vi "MyrioProject.vi"() -> ()   [LabVIEW 2018]
doc: "The myRIO Project template acquires acceleration data from the onboard accelerometer and displays the changes of acceleration values in a waveform chart."
uses:
  <vilib>/Platform/TimedLoop/XDataNode/timing_clust.ctl
  <vilib>/Platform/TimedLoop/XDataNode/nitl_modes.ctl
  <vilib>/Platform/TimedLoop/XDataNode/wakeup.ctl
  <vilib>/myRIO/Common/Instrument Driver Framework/myRIO v1.0/Encoder/typedefs/Encoder Signal Mode.ctl
  <vilib>/Analysis/Matrix/Datatypes/RealMatrix.ctl
  <vilib>/myRIO/Instrument Drivers/Onboard IO/PWM/typedefs/PWM Reference.ctl
  <vilib>/myRIO/Common/Instrument Driver Framework/Utilities/typedefs/myRIO Generic Hardware Reference.ctl
  <vilib>/myRIO/Common/Instrument Driver Framework/Utilities/typedefs/Hardware Version Enum.ctl
  <vilib>/myRIO/Common/Instrument Driver Framework/Utilities/typedefs/myRIO v1.0 Reference.ctl
  <vilib>/myRIO/Common/Instrument Driver Framework/Utilities/typedefs/Generic FPGA Reference.ctl
  <vilib>/myRIO/Common/Instrument Driver Framework/myRIO v1.0/PWM/typedefs/PWM Channels Enum.ctl
  <vilib>/myRIO/Instrument Drivers/Onboard IO/PWM/typedefs/PWM Configuration.ctl
  <vilib>/userdefined/High Color/nirio_resource_hc.ctl
  <vilib>/myRIO/Common/Instrument Driver Framework/myRIO v1.0/Encoder/typedefs/Encoder Configuration v1.0.ctl
  <vilib>/myRIO/Instrument Drivers/Onboard IO/Encoder/typedefs/Encoder Reference.ctl
  <vilib>/myRIO/Common/Instrument Driver Framework/myRIO v1.0/Encoder/typedefs/Encoder Channels Enum.ctl
  <vilib>/myRIO/Instrument Drivers/Onboard IO/DIO/typedefs/DIO Reference.ctl
  <vilib>/myRIO/Common/Instrument Driver Framework/myRIO v1.0/DIO/typedefs/DIO Channels List.ctl
  <vilib>/myRIO/Common/Instrument Driver Framework/myRIO v1.0/DIO/typedefs/DIO Channels Enum.ctl
  <vilib>/myRIO/Instrument Drivers/Onboard IO/AI/typedefs/AI Reference.ctl
  <vilib>/myRIO/Common/Instrument Driver Framework/myRIO v1.0/AI/typedefs/AI Channels List.ctl
  <vilib>/myRIO/Common/Instrument Driver Framework/myRIO v1.0/AI/typedefs/AI Channels Enum.ctl
  <vilib>/myRIO/Common/Instrument Driver Framework/Utilities/typedefs/Analog Scaling Constants List.ctl
  <vilib>/myRIO/Common/Instrument Driver Framework/Utilities/typedefs/Analog Scaling Constants.ctl
  <vilib>/myRIO/Common/Instrument Driver Framework/myRIO v1.0/PWM/vis/myRIO v1.1 Open PWM.vi
  <vilib>/myRIO/Common/Instrument Driver Framework/myRIO v1.0/Encoder/vis/myRIO v1.1 Open Encoder.vi
  <vilib>/myRIO/Common/Instrument Driver Framework/Utilities/vis/Is FPGA Ref Available.vi
  <vilib>/myRIO/Common/Instrument Driver Framework/myRIO v1.0/AI/vis/myRIO v1.1 Open AI.vi
  <vilib>/myRIO/Common/Instrument Driver Framework/myRIO v1.0/DIO/vis/myRIO v1.1 Open DIO.vi
  <vilib>/myRIO/Instrument Drivers/Onboard IO/PWM/vis/Set Duty Cycle and Frequency.vi
  <vilib>/myRIO/Instrument Drivers/Onboard IO/DIO/vis/Write.vi
  <vilib>/myRIO/Common/Instrument Driver Framework/Utilities/vis/Validate Channels.vi
  <vilib>/myRIO/Common/Instrument Driver Framework/myRIO v1.0/PWM/vis/myRIO v1.0 Reserve PWM.vi
  <vilib>/myRIO/Common/Instrument Driver Framework/myRIO v1.0/Encoder/vis/myRIO v1.0 Reserve Encoder.vi
  <vilib>/myRIO/Common/Instrument Driver Framework/myRIO v1.0/AI/vis/myRIO v1.0 Reserve AI.vi
  <vilib>/myRIO/Common/Instrument Driver Framework/myRIO v1.0/DIO/vis/myRIO v1.0 Reserve DIO.vi
  <vilib>/myRIO/Common/Instrument Driver Framework/myRIO v1.0/Encoder/vis/myRIO v1.0 Close Encoder.vi
  <vilib>/myRIO/Common/Instrument Driver Framework/myRIO v1.0/PWM/vis/myRIO v1.0 Close PWM.vi
  <vilib>/myRIO/Common/Instrument Driver Framework/myRIO v1.0/PWM/vis/myRIO v1.0 Build MUX Configuration PWM.vi
  <vilib>/myRIO/Common/Instrument Driver Framework/myRIO v1.0/Resource Manager/vis/myRIO v1.0 Reserve Channel List.vi
  <vilib>/myRIO/Common/Instrument Driver Framework/myRIO v1.0/Encoder/vis/myRIO v1.0 Build MUX Configuration Encoder.vi
  <vilib>/myRIO/Common/Instrument Driver Framework/myRIO v1.0/AI/vis/myRIO v1.0 Build MUX Configuration AI.vi
  <vilib>/myRIO/Common/Instrument Driver Framework/myRIO v1.0/DIO/vis/myRIO v1.0 Build MUX Configuration DIO.vi
  <vilib>/myRIO/Common/Instrument Driver Framework/myRIO v1.0/Encoder/vis/myRIO v1.0 Unreserve Encoder.vi
  <vilib>/myRIO/Common/Instrument Driver Framework/myRIO v1.0/PWM/vis/myRIO v1.0 Unreserve PWM.vi
  <vilib>/myRIO/Common/Instrument Driver Framework/myRIO v1.0/Resource Manager/vis/myRIO v1.0 Create Configuration List.vi
  <vilib>/myRIO/Common/Instrument Driver Framework/myRIO v1.0/Resource Manager/vis/myRIO v1.0 Reserve Channel.vi
  <vilib>/myRIO/Common/Instrument Driver Framework/myRIO v1.0/Resource Manager/vis/myRIO v1.0 Unreserve Channel.vi
  <vilib>/myRIO/Common/Instrument Driver Framework/myRIO v1.0/Resource Manager/vis/myRIO v1.0 Unreserve Channel List.vi
  <vilib>/myRIO/Common/Instrument Driver Framework/myRIO v1.0/Resource Manager/vis/myRIO v1.0 Build Mutex Name.vi
  <vilib>/Utility/VariantDataType/GetNumericInfo.vi
  <vilib>/Utility/error.llb/Error Cluster From Error Code.vi
  <vilib>/myRIO/Common/Instrument Driver Framework/myRIO v1.0/myRIO v1.1 Open.vi
  <vilib>/myRIO/Common/Instrument Driver Framework/Utilities/vis/IO Manager.vi
  <vilib>/myRIO/Common/Instrument Driver Framework/Utilities/vis/Configuration Manager.vi
  <vilib>/myRIO/Common/Instrument Driver Framework/myRIO v1.0/Resource Manager/vis/myRIO v1.0 Configure IO.vi
  <vilib>/myRIO/Common/Instrument Driver Framework/myRIO v1.0/myRIO v1.0 Close.vi
  <vilib>/myRIO/Common/Instrument Driver Framework/myRIO v1.0/PWM/vis/myRIO v1.0 Write PWM.vi
  <vilib>/myRIO/Common/Instrument Driver Framework/myRIO v1.0/Encoder/vis/myRIO v1.0 Configure Encoder.vi
  <vilib>/myRIO/Common/Instrument Driver Framework/myRIO v1.0/Encoder/vis/myRIO v1.0 Enable Encoder.vi
  <vilib>/myRIO/Common/Instrument Driver Framework/myRIO v1.0/DIO/vis/myRIO v1.0 Read DIO.vi
  <vilib>/myRIO/Common/Instrument Driver Framework/myRIO v1.0/AI/vis/myRIO v1.0 Get Scaling Constants AI.vi
  <vilib>/myRIO/Common/Instrument Driver Framework/myRIO v1.0/AI/vis/myRIO v1.0 Read AI.vi
  <vilib>/myRIO/Common/Instrument Driver Framework/myRIO v1.0/Encoder/vis/myRIO v1.0 Read Encoder.vi
  <vilib>/myRIO/Common/Instrument Driver Framework/myRIO v1.0/DIO/vis/myRIO v1.0 Write DIO.vi
  <vilib>/myRIO/Common/Instrument Driver Framework/myRIO v1.0/Encoder/vis/myRIO v1.0 Shutdown Encoder.vi
  <vilib>/myRIO/Common/Instrument Driver Framework/myRIO v1.0/PWM/vis/myRIO v1.0 Shutdown PWM.vi
  <vilib>/platform/TimedLoop/XDataNode/XDataNode.xnode
  <vilib>/myRIO/Instrument Drivers/Onboard IO/PWM/vis/myRIO PWM Open.xnode
  <vilib>/myRIO/Instrument Drivers/Onboard IO/Encoder/vis/myRIO Encoder Open.xnode
  <vilib>/myRIO/Express VI/Onboard IO/PWM/PWM Express VI.xnode
  <vilib>/myRIO/Express VI/Onboard Devices/Button/Button Express VI.xnode
  <vilib>/myRIO/Instrument Drivers/Onboard IO/DIO/vis/myRIO DIO Open.xnode
  <vilib>/myRIO/Express VI/Onboard IO/AI/AI Express VI.xnode
  <vilib>/myRIO/Instrument Drivers/Onboard IO/AI/vis/myRIO AI Open.xnode
  <vilib>/myRIO/Express VI/Onboard IO/DO/DO Express VI.xnode
  <vilib>/Platform/TimedLoop/XDataNode/XDNodeRunTimeDep.lvlib
  <vilib>/myRIO/Instrument Drivers/Onboard IO/Encoder/Encoder.lvlib
  <vilib>/myRIO/Instrument Drivers/Onboard IO/PWM/PWM.lvlib
  <vilib>/myRIO/Instrument Drivers/Onboard IO/DIO/DIO.lvlib
  <vilib>/myRIO/Instrument Drivers/Onboard IO/AI/AI.lvlib
  <vilib>/Analysis/Matrix/NI_Matrix.lvlib
panel:
  out "data":dbl
  out "Double 2":dbl
  out "Double":dbl
  out "sensor2 (A/AI2 (Pin 7))":dbl
  out "sensor1":dbl
  out "stallRojo (A/AI0 (Pin 3))":dbl
  out "stallBlanco (A/AI1 (Pin 5))":dbl
  in  "MANUAL 2":bool
  in  "Stop Button":bool
  in  "Start":bool
  out "element":dbl
  out "element 2":dbl
  out "subarray 2":dbl[][](array[numeric])
  out "subarray":dbl[][](array[numeric])
  out "vectores":dbl[][][](array[numeric])
  in  "saturacion":dbl=0.3
  in  "Duty Cycle 2":dbl(slide)=0.5 scale=0.05..0.1
  in  "Duty Cycle":dbl(slide)=0.5 scale=0.05..0.1
  in  "Reset Counter 2":bool
  in  "Reset Counter":bool
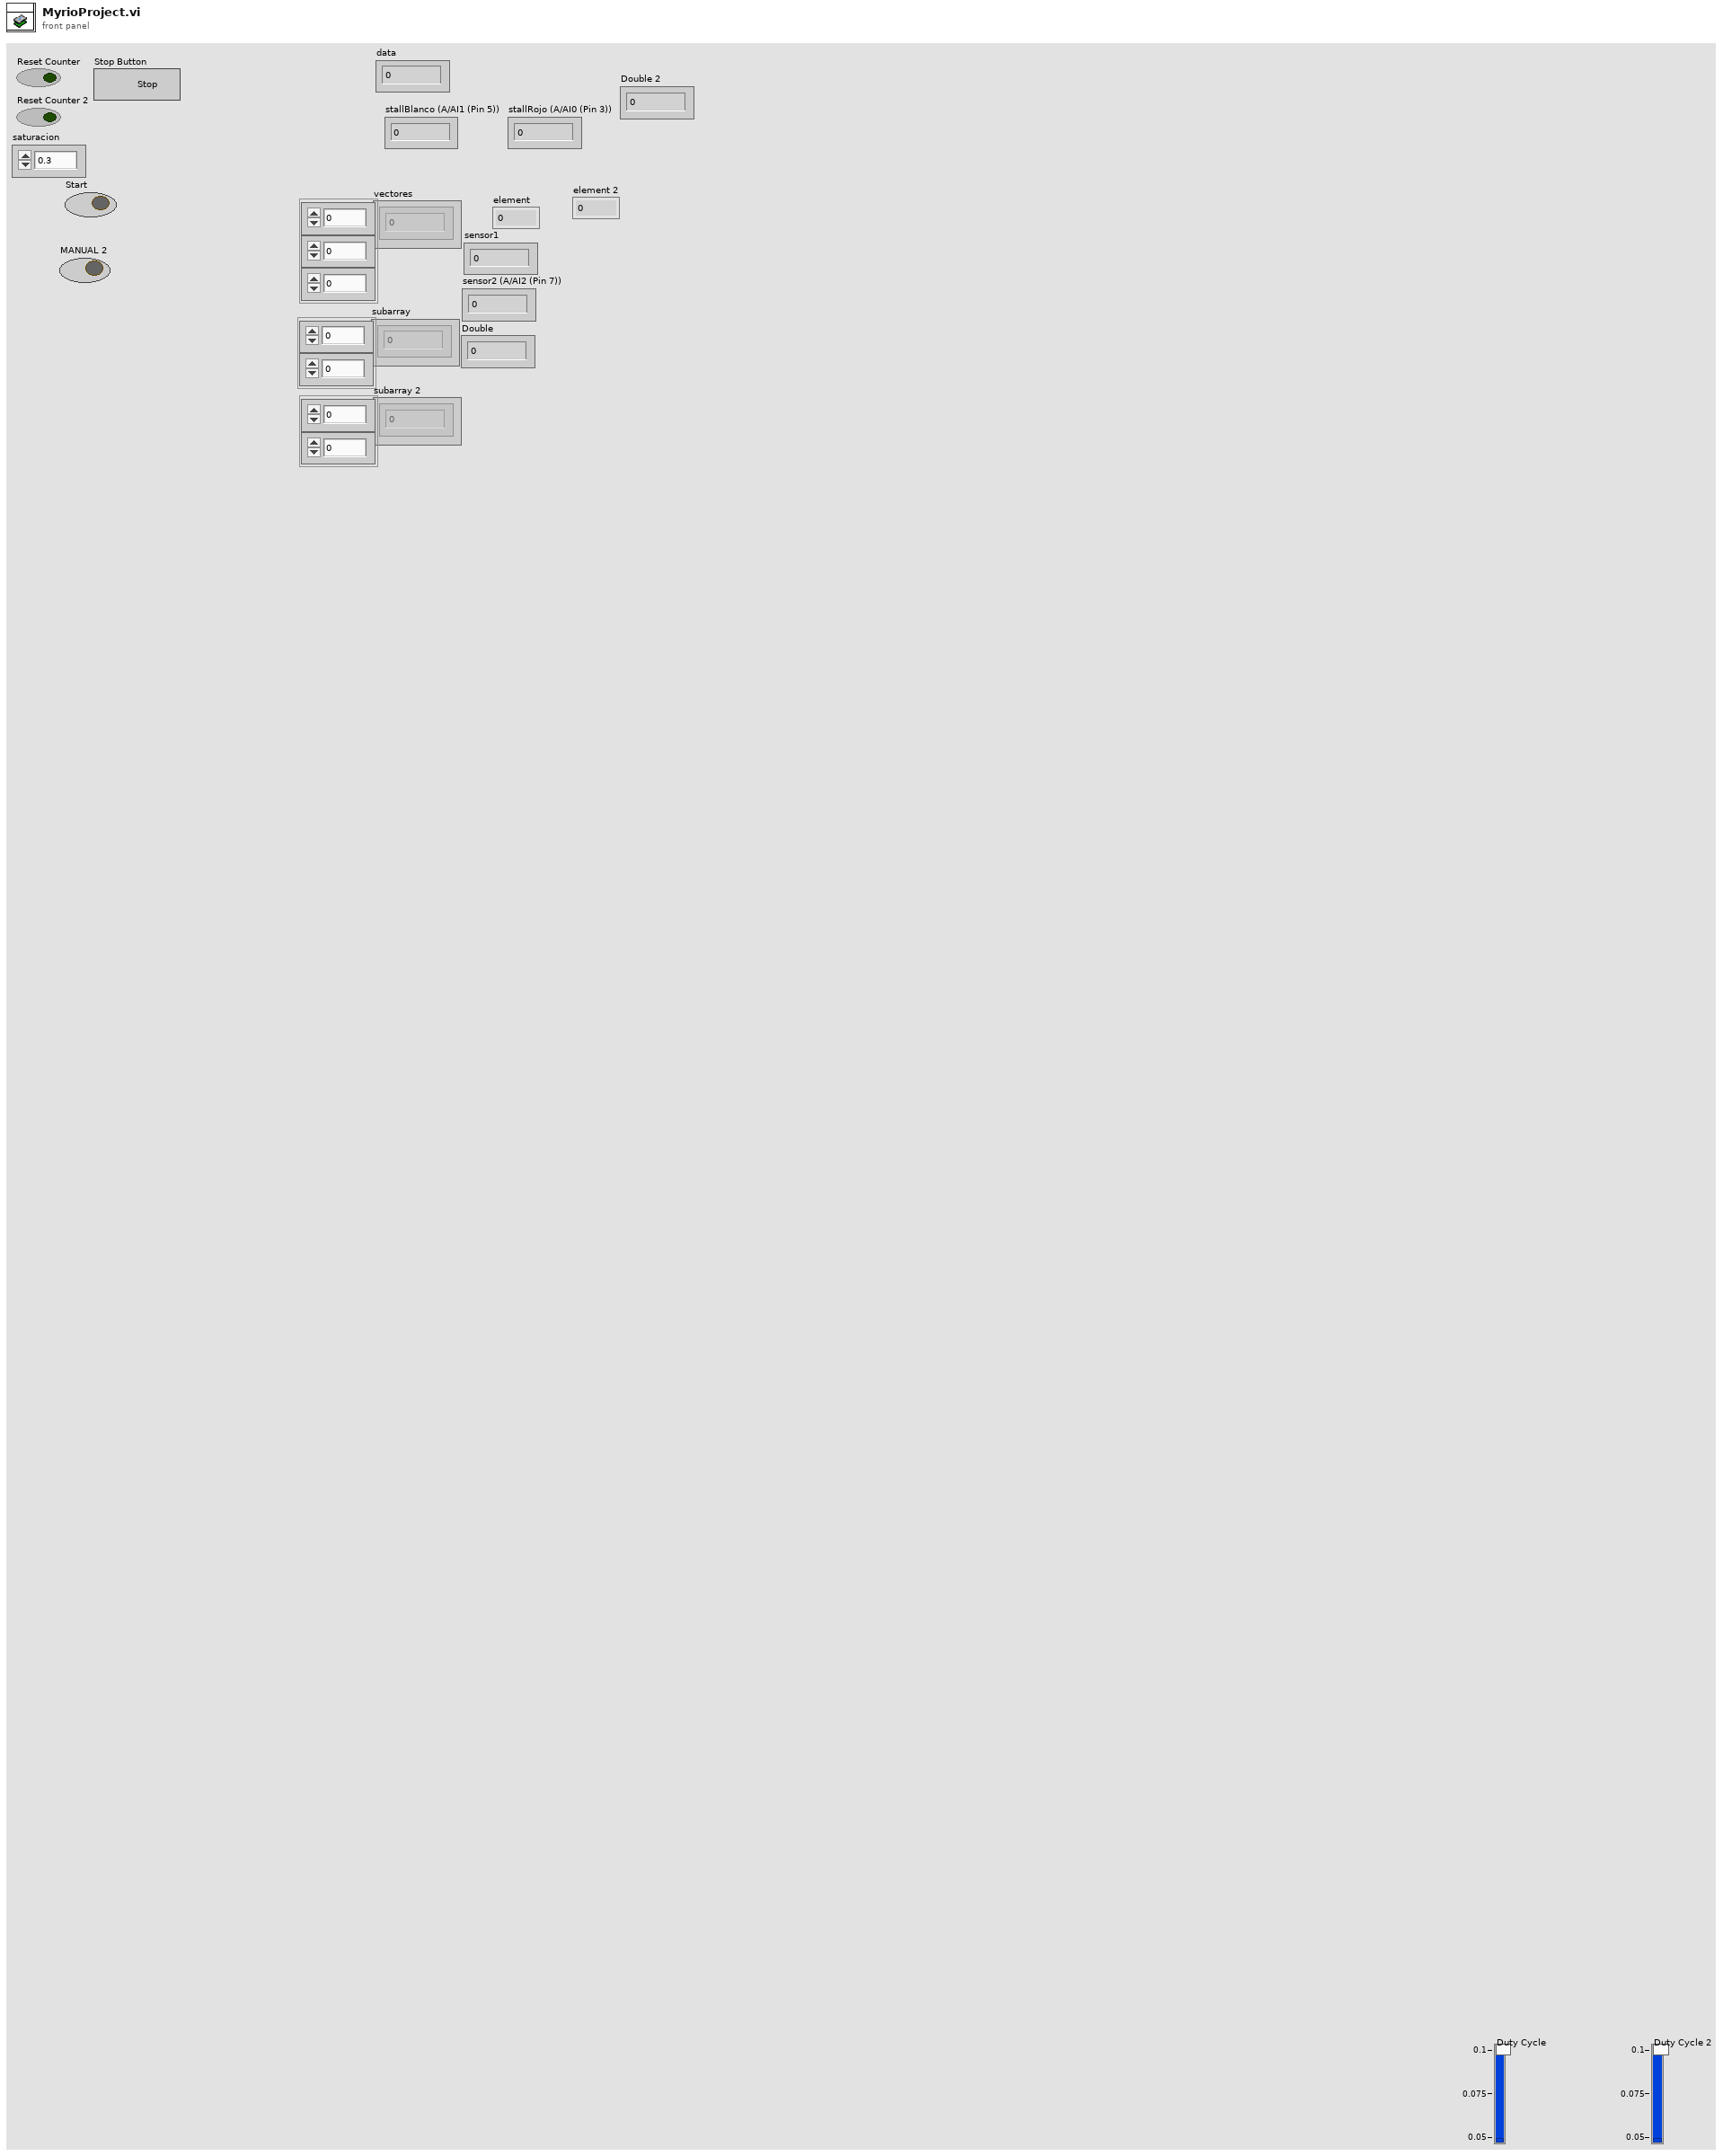
[diagram p1: front panel]
types:
  T1 = typedef "NI_Matrix.lvlib/RealMatrix.ctl" = dbl[][]
  T2 = typedef "Encoder Signal Mode.ctl" = enum16{"Quadrature phase signal", "Step and direction signal"}
  T3 = typedef "PWM.lvlib/PWM Reference.ctl" = cluster{"myRIO Reference":T4, "PWM Channels Enum":T8, "PWM Configuration":T9}
  T4 = typedef "myRIO Generic Hardware Reference.ctl" = cluster{"myRIO Model":T5, "myRIO Hardware Reference":T6}
  T5 = typedef "Hardware Version Enum.ctl" = enum16{"Unknown", "myRIO-1900", "myRIO-1950", "roboRIO", "NI ELVIS RIO CM", "ELVIS III"}
  T6 = typedef "myRIO v1.0 Reference.ctl" = cluster{"Generic FPGA Reference":T7, "Allow multiple opens":bool}
  T7 = typedef "Generic FPGA Reference.ctl" = refnum<k20>
  T8 = typedef "PWM Channels Enum.ctl" = enum16{"Not Connected", "C/PWM0", "C/PWM1", "A/PWM0", "A/PWM1", "A/PWM2", "A/PWM3", "A/PWM4", "A/PWM5", "A/PWM6", "A/PWM7", "A/PWM8", "A/PWM9", "A/PWM10", "A/PWM11", "A/PWM12", "A/PWM13", "A/PWM14", "A/PWM15", "A/PWM16", "A/PWM17", "A/PWM18", "A/PWM19", "B/PWM0", "B/PWM1", "B/PWM2", "B/PWM3", "B/PWM4", "B/PWM5", "B/PWM6", "B/PWM7", "B/PWM8", "B/PWM9", "B/PWM10", "B/PWM11", "B/PWM12", "B/PWM13", "B/PWM14", "B/PWM15", "B/PWM16", "B/PWM17", "B/PWM18", "B/PWM19", "PWM/PWM0", "PWM/PWM1", "PWM/PWM2", "PWM/PWM3", "PWM/PWM4", "PWM/PWM5", "PWM/PWM6", "PWM/PWM7", "PWM/PWM8", "PWM/PWM9"}
  T9 = typedef "PWM.lvlib/PWM Configuration.ctl" = cluster{"Frequency":dbl, "Duty Cycle":dbl}
  T10 = typedef "Encoder.lvlib/Encoder Reference.ctl" = cluster{"myRIO Reference":T4, "Encoder Channels Enum":T11}
  T11 = typedef "Encoder Channels Enum.ctl" = enum16{"Not Connected", "C/ENC0", "C/ENC1", "A/ENC", "A/ENC0", "A/ENC1", "A/ENC2", "A/ENC3", "A/ENC4", "A/ENC5", "A/ENC6", "A/ENC7", "A/ENC8", "A/ENC9", "B/ENC", "B/ENC0", "B/ENC1", "B/ENC2", "B/ENC3", "B/ENC4", "B/ENC5", "B/ENC6", "B/ENC7", "B/ENC8", "B/ENC9", "DIO/ENC0", "DIO/ENC1", "DIO/ENC2", "DIO/ENC3", "DIO/ENC4"}
  T12 = typedef "XDNodeRunTimeDep.lvlib/timing_clust.ctl" = cluster{"Expected End [f-1]":u64, "Actual End [f-1]":u64, "Finished Late? [f-1]":bool, "Expected End [i-1]":u64, "Actual End [i-1]":u64, "Finished Late? [i-1]":bool, "Expected Start [i]":u64, "Actual Start [i]":u64, "Expected Start [f]":u64, "Actual Start [f]":u64, "Source Name":string, "Structure Name":string, "Period":i64, "Deadline":i64, "Offset":i64, "Start":i64, "Priority":i32, "Timeout":i32, "Mode":T13, "Wakeup Reason":T14, "Error":errorcluster, "Source Type":string, "Secondary Source Type":string, "Global End Time":u64, "Global Start Time":u64, "Frame Duration":u64, "Iteration Duration":u64, "Assigned CPU":i32, "I/O Scan Engine Mode":u32}
  T13 = typedef "XDNodeRunTimeDep.lvlib/nitl_modes.ctl" = enum32{"No Change", "Process missed periods, maintain original phase", "Discard missed periods, maintain original phase", "Process missed periods, ignore original phase", "Discard missed periods, ignore original phase"}
  T14 = typedef "XDNodeRunTimeDep.lvlib/wakeup.ctl" = enum32{"Normal", "Aborted", "Asynchronous wakeup", "Timing source error", "Timed loop error", "Timeout"}
  T15 = enum16{"normal", "grande-Sensor", "grande home", "peque-sensor", "peque- home", "peque-reset"}
  T16 = typedef "nirio_resource_hc.ctl" = tag
  T17 = typedef "AI.lvlib/AI Reference.ctl" = cluster{"myRIO Reference":T4, "AI Channels List":T18, "AI Scaling Constants List":T20}
  T18 = typedef "AI Channels List.ctl" = T19[]
  T19 = typedef "AI Channels Enum.ctl" = enum16{"Not Connected", "AudioIn/Left", "AudioIn/Right", "C/AI0", "C/AI1", "A/AI0", "A/AI1", "A/AI2", "A/AI3", "A/AI4", "A/AI5", "A/AI6", "A/AI7", "B/AI0", "B/AI1", "B/AI2", "B/AI3", "B/AI4", "B/AI5", "B/AI6", "B/AI7", "AI/AI0", "AI/AI1", "AI/AI2", "AI/AI3", "A/AI0 (DIFF)", "A/AI1 (DIFF)", "A/AI2 (DIFF)", "A/AI3 (DIFF)", "B/AI0 (DIFF)", "B/AI1 (DIFF)", "B/AI2 (DIFF)", "B/AI3 (DIFF)"}
  T20 = typedef "Analog Scaling Constants List.ctl" = T21[]
  T21 = typedef "Analog Scaling Constants.ctl" = cluster{"LSB Weight (Volts)":dbl, "Offset (Volts)":dbl, "Signed?":bool}
  T22 = typedef "DIO.lvlib/DIO Reference.ctl" = cluster{"myRIO Reference":T4, "DIO Channels List":T23}
  T23 = typedef "DIO Channels List.ctl" = T24[]
  T24 = typedef "DIO Channels Enum.ctl" = enum16{"Not Connected", "C/DIO0", "C/DIO1", "C/DIO2", "C/DIO3", "C/DIO4", "C/DIO5", "C/DIO6", "C/DIO7", "A/DIO0", "A/DIO1", "A/DIO2", "A/DIO3", "A/DIO4", "A/DIO5", "A/DIO6", "A/DIO7", "A/DIO8", "A/DIO9", "A/DIO10", "A/DIO11", "A/DIO12", "A/DIO13", "A/DIO14", "A/DIO15", "A/DIO16", "A/DIO17", "A/DIO18", "A/DIO19", "B/DIO0", "B/DIO1", "B/DIO2", "B/DIO3", "B/DIO4", "B/DIO5", "B/DIO6", "B/DIO7", "B/DIO8", "B/DIO9", "B/DIO10", "B/DIO11", "B/DIO12", "B/DIO13", "B/DIO14", "B/DIO15", "B/DIO16", "B/DIO17", "B/DIO18", "B/DIO19", "LED0", "LED1", "LED2", "LED3", "Button0", "DIO/DIO0", "DIO/DIO1", "DIO/DIO2", "DIO/DIO3", "DIO/DIO4", "DIO/DIO5", "DIO/DIO6", "DIO/DIO7", "DIO/DIO8", "DIO/DIO9", "SPI/CS0", "SPI/CS1", "SPI/CS2", "SPI/CS3", "LED RADIO (Green)", "LED RADIO (Red)", "LED COMM (Green)", "LED COMM (Red)", "LED MODE (Green)", "LED MODE (Red)"}
  T25 = cluster{dbl, "saturacion":dbl, "Counter Value":i32, "seconds since 1Jan1904":timestamp, dbl, dbl, dbl}
  T26 = cluster{"Double":dbl, "dbl Scaled Value":dbl, "Output":dbl, "seconds since 1Jan1904":timestamp, dbl, dbl, dbl}
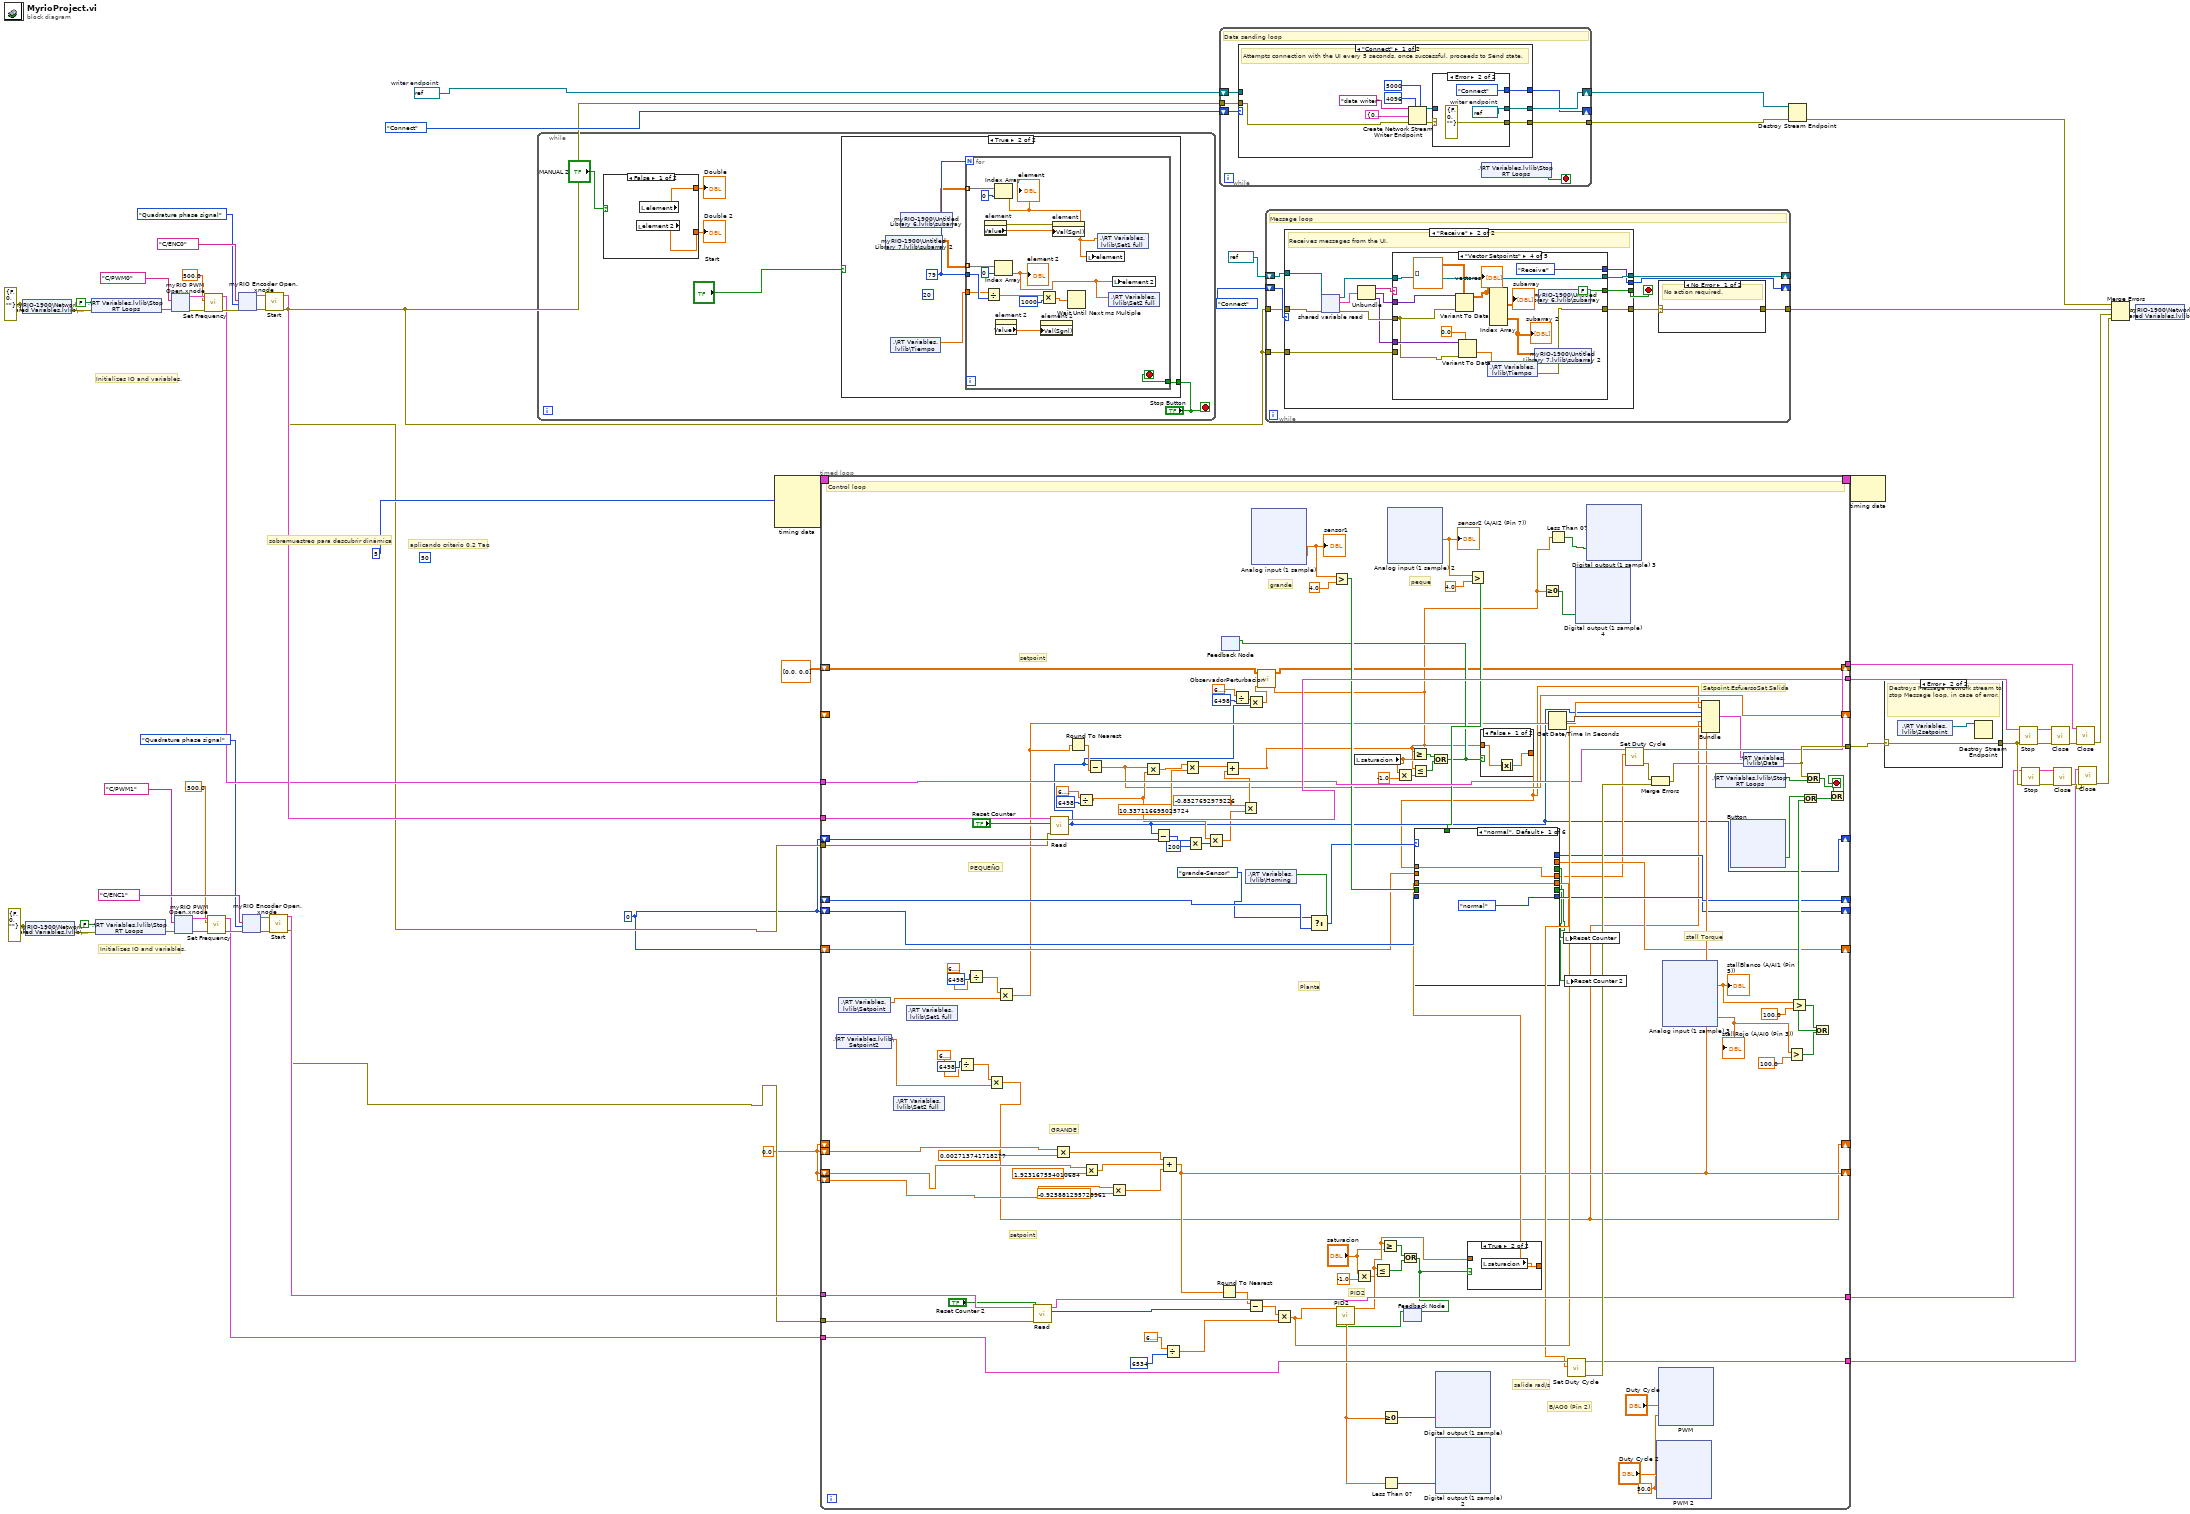
[diagram p0: block diagram]
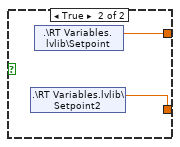
[diagram p2: hidden frame]
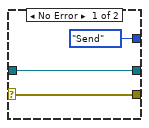
[diagram p5: hidden frame]
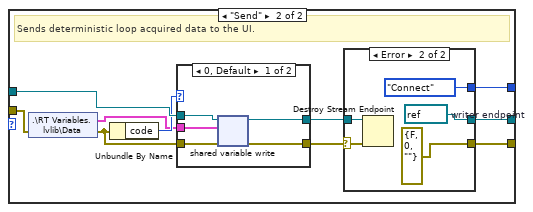
[diagram p6: hidden frame]
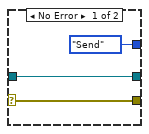
[diagram p7: hidden frame]
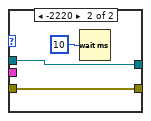
[diagram p8: hidden frame]
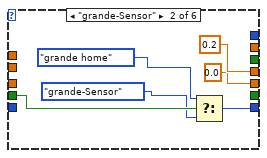
[diagram p9: hidden frame]
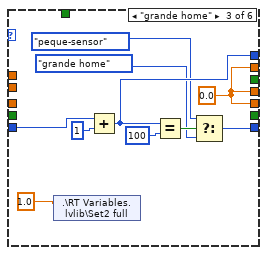
[diagram p10: hidden frame]
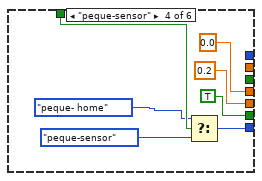
[diagram p11: hidden frame]
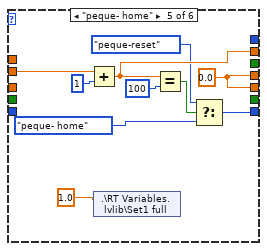
[diagram p12: hidden frame]
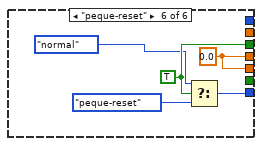
[diagram p13: hidden frame]
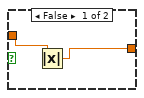
[diagram p14: hidden frame]
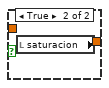
[diagram p15: hidden frame]
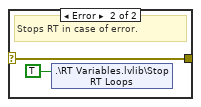
[diagram p16: hidden frame]
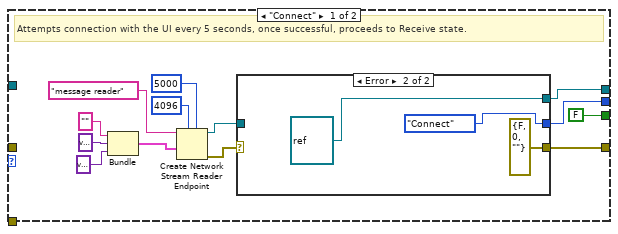
[diagram p17: hidden frame]
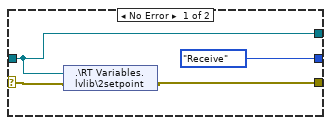
[diagram p18: hidden frame]
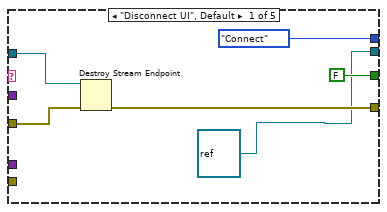
[diagram p19: hidden frame]
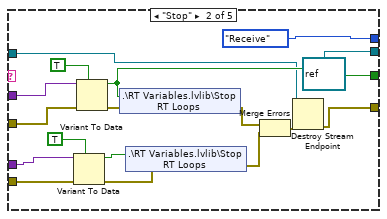
[diagram p20: hidden frame]
diagram:
  w2 = 0.0
  w3 = 0
  (unwired) 50
  w15 = refnum<k21> refnum  # writer endpoint
  w28 = errorcluster {"status"=FALSE, "code"=0, "source"=""} ("error IO")
  w50 = errorcluster {"status"=FALSE, "code"=0, "source"=""} ("error IO")
  # "aplicando criterio 0.2 Tao"
  # "sobremuestreo para descubrir dinámica"
  # "Initializes IO and variables."
  # "Initializes IO and variables."
  n1 = shared-variable "myRIO-1900\\Network Shared Variables.lvlib\\error IO"(w50, error in=w50) -> (error out=w51:errorcluster)
  n2 = shared-variable "myRIO-1900\\Network Shared Variables.lvlib\\error IO"(w28, error in=w28) -> (error out=w29:errorcluster)
  n3 = shared-variable ".\\RT Variables.lvlib\\Stop RT Loops"(FALSE ("Stop RT Loops"), error in=w51) -> (error out=w38:errorcluster)
  n4 = shared-variable ".\\RT Variables.lvlib\\Stop RT Loops"(FALSE ("Stop RT Loops"), error in=w29) -> (error out=w21:errorcluster)
  n5 = xnode "myRIO PWM Open.xnode"("error in (no error)"=w38, "Channel Name"=tag "C/PWM0") -> ("error out"=w40:errorcluster, "PWM Ref Out"=w39:T3)  [unwired: 1 in]
  n6 = xnode "myRIO PWM Open.xnode"("error in (no error)"=w21, "Channel Name"=tag "C/PWM1") -> ("error out"=w23:errorcluster, "PWM Ref Out"=w22:T3)  [unwired: 1 in]
  n7 = call <vilib>:"Set Frequency.vi"("error in (no error)"=w40, "Frequency [Hz]"=500.0, "PWM Ref In"=w39) -> ("error out"=w37:errorcluster, "PWM Ref Out"=w34:T3)  [unwired: 6 in]
  n8 = call <vilib>:"Set Frequency.vi"("error in (no error)"=w23, "Frequency [Hz]"=500.0, "PWM Ref In"=w22) -> ("error out"=w20:errorcluster, "PWM Ref Out"=w16:T3)  [unwired: 6 in]
  n9 = xnode "myRIO Encoder Open.xnode"("error in (no error)"=w37, "Channel Name"=tag "C/ENC0", "Encoder Signal Mode"=Encoder_Signal_Mode."Quadrature phase signal") -> ("error out"=w47:errorcluster, "Encoder Ref Out"=w46:T10)  [unwired: 2 in]
  n10 = xnode "myRIO Encoder Open.xnode"("error in (no error)"=w20, "Channel Name"=tag "C/ENC1", "Encoder Signal Mode"=Encoder_Signal_Mode."Quadrature phase signal") -> ("error out"=w26:errorcluster, "Encoder Ref Out"=w25:T10)  [unwired: 2 in]
  n11 = call <vilib>:"Start.vi"("error in (no error)"=w47, "Encoder Ref In"=w46) -> ("error out"=w5:errorcluster, "Encoder Ref Out"=w44:T10)  [unwired: 8 in]
  n12 = call <vilib>:"Start.vi"("error in (no error)"=w26, "Encoder Ref In"=w25) -> ("error out"=w4:errorcluster, "Encoder Ref Out"=w17:T10)  [unwired: 8 in]
  n13 = while {
    stop <- "Stop Button" stop-if-true
    n14 = case shown="False" "MANUAL 2" {
      tunnel: [w68 w70] -> w62
      tunnel: [w67 w69] -> w63
      frame False {
        n15 = local read "element 2"() -> (w68:dbl)
        n16 = local read "element"() -> (w67:dbl)
      }
      frame True {
        n17 = shared-variable ".\\RT Variables.lvlib\\Setpoint2"() -> (w70:dbl)  [unwired: 1 in, 1 out]
        n18 = shared-variable ".\\RT Variables.lvlib\\Setpoint"() -> (w69:dbl)  [unwired: 1 in, 1 out]
      }
    }
    "Double" <- w63
    "Double 2" <- w62
    n19 = case shown="True" "Start" {
      tunnel: "Stop Button" -> [_ w72]
      frame False {
      }
      frame True {
        (unwired) 20
        w75 = 79
        n20 = shared-variable "myRIO-1900\\Untitled Library 7.lvlib\\subarray 2"() -> (w73:dbl[][])  [unwired: 1 in, 1 out]
        n21 = shared-variable ".\\RT Variables.lvlib\\Tiempo"() -> (w71:dbl)  [unwired: 1 in, 1 out]
        n22 = shared-variable "myRIO-1900\\Untitled Library 6.lvlib\\subarray"() -> (w74:dbl[][])  [unwired: 1 in, 1 out]
        n23 = for {
          N: w75 -> [_]
          tunnel: w75 -> [w88]
          tunnel: w74 -> [w87] mode=indexing
          tunnel: w71 -> [w85]
          tunnel: w73 -> [w83] mode=indexing
          tunnel: w72 -> [w78]
          stop <- w78 stop-if-true
          n24 = property on="element" class="DigNum (strict)"() -> (error out=w81:errorcluster, "Value"=w82:dbl)  [unwired: 2 in, 1 out]
          n25 = Divide(x=w85, y=w88) -> (x/y=w90:dbl)
          n26 = Index Array(array=w87, index=0) -> (element=w77:dbl)
          "element" <- w77
          n27 = Index Array(array=w83, index=0) -> (element=w76:dbl)
          "element 2" <- w76
          n28 = property on="element 2" class="DigNum (strict)"() -> ("Value"=w80:dbl)  [unwired: 2 in, 2 out]
          n29 = Multiply(x=w90, y=1000) -> (x*y=w79:dbl)
          n30 = property on="element 2" class="DigNum (strict)"("Val(Sgnl)"=w80) -> ()  [unwired: 2 in, 2 out]
          n31 = property on="element" class="DigNum (strict)"(error in=w81, "Val(Sgnl)"=w82) -> ()  [unwired: 1 in, 2 out]
          n32 = Wait Until Next ms Multiple(millisecond multiple=w79) -> ()  [unwired: 1 out]
          n33 = local write "element"(w77) -> ()
          n34 = shared-variable ".\\RT Variables.lvlib\\Set1 full"(w77) -> ()  [unwired: 1 in, 1 out]
          n35 = shared-variable ".\\RT Variables.lvlib\\Set2 full"(w76) -> ()  [unwired: 1 in, 1 out]
          n36 = local write "element 2"(w76) -> ()
        }
      }
    }
  }
  n37 = node-c288(i64 5 ("Period")) -> (w61:T12)  [unwired: 3 in]
  n38 = timed-loop {
    timing: w61 -> [_]
    timing-out: [_] -> w60
    tunnel: [w210] -> w49
    tunnel: w44 -> [w173]
    tunnel: [w172] -> w41
    tunnel: w34 -> [w161]
    tunnel: [w209] -> w33
    tunnel: w17 -> [w206]
    tunnel: w16 -> [w205]
    tunnel: [w201] -> w10
    tunnel: [w200] -> w9
    shift-right: [w127] -> _
    shift-left: w2 -> [_]
    shift-left: w2 -> [w187]
    shift-right: [w177] -> _
    shift-left: w2 -> [w186]
    shift-left: w2 -> [w185]
    shift-right: [w160] -> _
    shift-left: _ -> [w159]
    shift-right: [w157] -> _
    shift-left: w3 -> [w156]
    shift-right: [w152] -> _
    shift-left: w3 -> [w151]
    shift-right: [w100] -> _
    shift-left: w3 -> [w144]
    tunnel: w4 -> [w139]
    tunnel: w5 -> [w138]
    shift-right: [w99] -> _
    shift-left: T1 [[0.0], [0.0]] ("xk +1") -> [w106]
    shift-right: [w96] -> _
    shift-left: _ -> [_]
    stop <- w198 stop-if-true
    w141 = 50.0 ("Frequency [Hz]")
    # "setpoint"
    # "PEQUEÑO"
    # "peque"
    # "grande"
    # "stall Torque"
    # "Setpoint,EsfuersoSat,Salida"
    # "setpoint"
    # "PID2"
    # "GRANDE"
    # "Planta"
    # "salida rad/s"
    # "B/AO0 (Pin 2)"
    # "Control loop"
    n39 = shared-variable ".\\RT Variables.lvlib\\Setpoint2"() -> (w109:dbl)  [unwired: 1 in, 1 out]
    n40 = shared-variable ".\\RT Variables.lvlib\\Setpoint"() -> (w108:dbl)  [unwired: 1 in, 1 out]
    n41 = shared-variable ".\\RT Variables.lvlib\\Set2 full"() -> ()  [unwired: 1 in, 2 out]
    n42 = shared-variable ".\\RT Variables.lvlib\\Set1 full"() -> ()  [unwired: 1 in, 2 out]
    n43 = Divide(x=6498, y=6.283185307179586) -> (x/y=w128:dbl)
    n44 = Divide(x=6498, y=6.283185307179586) -> (x/y=w131:dbl)
    n45 = Multiply(x=w128, y=w109) -> (x*y=w127:dbl)
    n46 = Multiply(x=w131, y=w108) -> (x*y=w107:dbl)
    n47 = call <vilib>:"Read.vi"("error in (no error)"=w139, "Reset Counter"="Reset Counter 2", "Encoder Ref In"=w206) -> ("Counter Value"=w181:i32, "Encoder Ref Out"=w201:T10)  [unwired: 4 in, 3 out]
    n48 = call <vilib>:"Read.vi"("error in (no error)"=w138, "Reset Counter"="Reset Counter", "Encoder Ref In"=w173) -> ("Counter Value"=w100:i32, "Encoder Ref Out"=w172:T10)  [unwired: 4 in, 3 out]
    n49 = Multiply(x=w187, y=0.002713741718277) -> (x*y=w189:dbl)
    n50 = Round To Nearest(number=w107) -> (nearest integer value=w171:dbl)
    n51 = Divide(x=6.283185307179586, y=6498) -> (x/y=w110:dbl)
    n52 = Multiply(x=w186, y=1.923167554010684) -> (x*y=w190:dbl)
    n53 = Subtract(x=w100, y=w171) -> (x-y=w96:dbl)
    n54 = Multiply(x=w185, y=-0.925881295728961) -> (x*y=w188:dbl)
    n55 = Multiply(x=w96, y=w110) -> (x*y=w115:dbl)
    n56 = Subtract(x=w100, y=w144) -> (x-y=w118:i32)
    n57 = Compound Arithmetic op=ADD(w189, w190, w188) -> (w177:dbl)
    n58 = Divide(x=6.283185307179586, y=6534) -> (x/y=w179:dbl)
    n59 = Multiply(x=w115, y=10.337116695025724) -> (x*y=w98:dbl)
    n60 = Multiply(x=w118, y=200) -> (x*y=w111:i32)
    n61 = Multiply(x=w110, y=w111) -> (x*y=w97:dbl)
    n62 = Round To Nearest(number=w177) -> (nearest integer value=w176:dbl)
    n63 = feedback #1() -> ()  [unwired: 2 in]
    n64 = Divide(x=6.283185307179586, y=6498) -> (x/y=w101:dbl)
    n65 = Multiply(x=-0.8527692979226, y=w97) -> (x*y=w145:dbl)
    n66 = Add(x=w98, y=w145) -> (x+y=w91:dbl)
    n67 = shared-variable ".\\RT Variables.lvlib\\Homing"() -> (w162:bool)  [unwired: 1 in, 1 out]
    n68 = Multiply(x=w101, y=w100) -> (x*y=w102:dbl)
    n69 = Subtract(x=w176, y=w181) -> (x-y=w180:dbl)
    n70 = xnode "Analog input (1 sample)"() -> ("A/AI3 (Pin 9)"=w135:dbl)  [unwired: 1 in, 1 out]
    "sensor1" <- w135
    n71 = call "ObservadorPerturbacion.vi"("entrada planta"=w91, "salida planta"=w102, "xk +1"=w106) -> ("xk"=w99:T1)  [unwired: 6 in, 2 out]
    n72 = Multiply(x=w180, y=w179) -> (x*y=w178:dbl)
    n73 = Select(t=T15."grande-Sensor" ("Enum"), s=w162, f=w159) -> (s? t:f=w112:T15)
    n74 = Greater?(x=w135, y=4.0) -> (0:w158:bool)
    n75 = local read "saturacion"() -> (w124:dbl)
    n76 = Multiply(x="saturacion", y=-1.0) -> (x*y=w123:dbl)
    n77 = xnode "Analog input (1 sample) 2"() -> ("sensor2 (A/AI2 (Pin 7))"=w134:dbl)  [unwired: 1 in, 1 out]
    "sensor2 (A/AI2 (Pin 7))" <- w134
    n78 = Multiply(x=w124, y=-1.0) -> (x*y=w126:dbl)
    n79 = feedback #2() -> (w183:bool)  [unwired: 1 in]
    n80 = call "PID2.vi"("Boolean"=w183, "Numeric in"=w178) -> ("Numeric out"=w184:dbl)  [unwired: 9 in]
    n81 = Less Or Equal?(x=w184, y=w123) -> (x <= y?=w194:bool)
    n82 = Greater Or Equal?(x=w184, y="saturacion") -> (x >= y?=w195:bool)
    n83 = Greater Or Equal To 0?(x=w184) -> (x >= 0?=w120:bool)
    n84 = Less Than 0?(x=w184) -> (x < 0?=w119:bool)
    n85 = Or(x=w195, y=w194) -> (x .or. y?=w182:bool)
    n86 = feedback-in #2(w182) -> ()
    n87 = Greater Or Equal?(x=w91, y=w124) -> (x >= y?=w197:bool)
    n88 = Less Or Equal?(x=w91, y=w126) -> (x <= y?=w196:bool)
    n89 = Or(x=w197, y=w196) -> (x .or. y?=w114:bool)
    n90 = feedback-in #1(w114) -> ()
    n91 = xnode "Digital output (1 sample)"("A/DIO0 (Pin 11)"=w120) -> ()  [unwired: 1 in, 1 out]
    n92 = xnode "Digital output (1 sample) 2"("A/DIO1 (Pin 13)"=w119) -> ()  [unwired: 1 in, 1 out]
    n93 = case shown="True" w182 {
      tunnel: [w576 w578] -> w155
      tunnel: w184 -> [w577 _]
      frame False {
        n94 = Absolute Value(x=w577) -> (abs(x)=w576:dbl)
      }
      frame True {
        n95 = local read "saturacion"() -> (w578:dbl)
      }
    }
    n96 = Greater?(x=w134, y=4.0) -> (0:w153:bool)
    n97 = case shown="False" w114 {
      tunnel: [w579 w581] -> w94
      tunnel: w91 -> [w580 _]
      frame False {
        n98 = Absolute Value(x=w580) -> (abs(x)=w579:dbl)
      }
      frame True {
        n99 = local read "saturacion"() -> (w581:dbl)
      }
    }
    n100 = case shown="\"normal\", Default" w112 {
      tunnel: w94 -> [w285 _ _ _ _ _]
      tunnel: [w285 0.2 ("f") w292 0.0 ("f") w309 w323] -> w105
      tunnel: [T15."normal" ("Enum") w289 w296 w306 w315 w321] -> w160
      tunnel: w158 -> [_ w290 _ _ _ _]
      tunnel: [_ _ w299 _ _ _] -> w157
      tunnel: w156 -> [_ _ w300 _ _ _]
      tunnel: w155 -> [w284 _ _ _ _ _]
      tunnel: [w284 0.0 ("f") w292 0.2 ("f") w309 w323] -> w154
      tunnel: w153 -> [_ _ _ w307 _ _]
      tunnel: [_ _ w292 _ w314 _] -> w152
      tunnel: w151 -> [_ _ _ _ w313 _]
      tunnel: [_ _ _ TRUE _ _] -> w149
      tunnel: [_ _ _ _ _ w320] -> w147
      frame "normal", Default {
      }
      frame "grande-Sensor" {
        n101 = Select(t=T15."grande home" ("Enum"), s=w290, f=T15."grande-Sensor" ("Enum")) -> (s? t:f=w289:T15)
      }
      frame "grande home" {
        w292 = 0.0
        n102 = shared-variable ".\\RT Variables.lvlib\\Set2 full"(1.0) -> ()  [unwired: 1 in, 1 out]
        n103 = Add(x=w300, y=1) -> (x+y=w299:i32)
        n104 = Equal?(x=w299, y=100) -> (x = y?=w297:bool)
        n105 = Select(t=T15."peque-sensor" ("Enum"), s=w297, f=T15."grande home" ("Enum")) -> (s? t:f=w296:T15)
      }
      frame "peque-sensor" {
        n106 = Select(t=T15."peque- home" ("Enum"), s=w307, f=T15."peque-sensor" ("Enum")) -> (s? t:f=w306:T15)
      }
      frame "peque- home" {
        w309 = 0.0 ("f")
        n107 = Add(x=w313, y=1) -> (x+y=w314:dbl)
        n108 = shared-variable ".\\RT Variables.lvlib\\Set1 full"(1.0) -> ()  [unwired: 1 in, 1 out]
        n109 = Equal?(x=w314, y=100) -> (x = y?=w318:bool)
        n110 = Select(t=T15."peque-reset" ("Enum"), s=w318, f=T15."peque- home" ("Enum")) -> (s? t:f=w315:T15)
      }
      frame "peque-reset" {
        w320 = TRUE
        w323 = 0.0 ("f")
        n111 = Select(t=T15."normal" ("Enum"), s=w320, f=T15."peque-reset" ("Enum")) -> (s? t:f=w321:T15)
      }
    }
    n112 = Greater Or Equal To 0?(x=w91) -> (x >= 0?=w93:bool)
    n113 = Get Date/Time In Seconds() -> (seconds since 1Jan1904=w212:timestamp)
    n114 = Less Than 0?(x=w91) -> (x < 0?=w92:bool)
    n115 = local write "Reset Counter"(w149) -> ()
    n116 = local write "Reset Counter 2"(w147) -> ()
    n117 = call <vilib>:"Set Duty Cycle.vi"("Duty Cycle"=w154, "PWM Ref In"=w205) -> ("error out"=w204:errorcluster, "PWM Ref Out"=w200:T3)  [unwired: 7 in]
    n118 = xnode "Digital output (1 sample) 4"("A/DIO3 (Pin 17)"=w93) -> ()  [unwired: 1 in, 1 out]
    n119 = xnode "Digital output (1 sample) 3"("A/DIO2 (Pin 15)"=w92) -> ()  [unwired: 1 in, 1 out]
    n120 = call <vilib>:"Set Duty Cycle.vi"("Duty Cycle"=w105, "PWM Ref In"=w161) -> ("error out"=w203:errorcluster, "PWM Ref Out"=w209:T3)  [unwired: 7 in]
    n121 = Merge Errors(w203, w204) -> (w202:errorcluster)
    n122 = xnode "PWM 2"("Duty Cycle"="Duty Cycle 2", "Frequency [Hz]"=w141) -> ()  [unwired: 1 in, 1 out]
    n123 = xnode "PWM"("Duty Cycle"="Duty Cycle", "Frequency [Hz]"=w141) -> ()  [unwired: 1 in, 1 out]
    n124 = xnode "Analog input (1 sample) 3"() -> ("stallBlanco (A/AI1 (Pin 5))"=w137:dbl, "stallRojo (A/AI0 (Pin 3))"=w136:dbl)  [unwired: 1 in, 1 out]
    "stallBlanco (A/AI1 (Pin 5))" <- w137
    "stallRojo (A/AI0 (Pin 3))" <- w136
    n125 = Bundle(w107, "saturacion"=w94, "Counter Value"=w100, "seconds since 1Jan1904"=w212, w127, w178, w177) -> (w95:T25)  [unwired: 1 in]
    n126 = shared-variable ".\\RT Variables.lvlib\\Stop RT Loops"() -> (w211:bool)  [unwired: 1 in, 1 out]
    n127 = xnode "Button"() -> ("Value"=w143:bool)  [unwired: 1 in, 1 out]
    n128 = shared-variable ".\\RT Variables.lvlib\\Data"(w95, error in=w202) -> (error out=w210:errorcluster)
    n129 = Greater?(x=w136, y=100.0) -> (0:w164:bool)
    n130 = Greater?(x=w137, y=100.0) -> (0:w165:bool)
    n131 = Or(x=w210, y=w211) -> (x .or. y?=w199:bool)
    n132 = Or(x=w165, y=w164) -> (x .or. y?=w166:bool)
    n133 = Or(x=w143, y=w166) -> (x .or. y?=w163:bool)
    n134 = Or(x=w199, y=w163) -> (x .or. y?=w198:bool)
  }
  n135 = while {
    shift-right: [w623] -> w56
    shift-left: w15 -> [w621]
    tunnel: [w622] -> w57
    tunnel: w5 -> [w620]
    shift-right: [w619] -> _
    shift-left: enum16{"Connect", "Send"}."Connect" ("Message states") -> [w624]
    stop <- w625 stop-if-true
    # "Data sending loop"
    n136 = case shown="\"Connect\"" w624 {
      tunnel: [w629 w644] -> w622
      tunnel: [w627 w642] -> w623
      tunnel: [w633 w645] -> w619
      tunnel: w621 -> [_ w651]
      tunnel: w620 -> [w630 w650]
      frame "Connect" {
        # "Attempts connection with the UI every 5 seconds, once successful, proceeds to Send state."
        n137 = Create Network Stream Writer Endpoint(5:5000 ("timeout in ms (-1)"), 7:4096 ("writer buffer size"), 8:w630, 9:T26 {"Double"=0.0, "dbl Scaled Value"=0.0, "Output"=0.0, "seconds since 1Jan1904"=timestamp(0 s since 1904-01-01), 0.0, 0.0, 0.0} ("Data"), 11:"data writer" ("writer name")) -> (0:w631:errorcluster, 3:w628:refnum<k21>)  [unwired: 2 in]
        n138 = case shown="Error" w631 {
          selector: w631 -> [w636 _]
          tunnel: [enum16{"Connect", "Send"}."Send" ("Message states") enum16{"Connect", "Send"}."Connect" ("Message states")] -> w633
          tunnel: [w636 errorcluster {"status"=FALSE, "code"=0, "source"=""} ("error IO")] -> w629
          tunnel: w628 -> [w638 _]
          tunnel: [w638 w639] -> w627
          frame No Error {
          }
          frame Error {
            w639 = refnum<k21> refnum  # writer endpoint
          }
        }
      }
      frame "Send" {
        # "Sends deterministic loop acquired data to the UI."
        n139 = shared-variable ".\\RT Variables.lvlib\\Data"(error in=w650) -> (w647:T26, error out=w649:errorcluster)
        n140 = Unbundle By Name(w649) -> ("code"=w648:i32)
        n141 = case shown="0, Default" w648 {
          tunnel: [w664 w666] -> w646
          tunnel: [w663 w665] -> w643
          tunnel: w651 -> [w662 w665]
          tunnel: w649 -> [w661 w666]
          tunnel: w647 -> [w660 _]
          frame 0, Default {
            n142 = shared-variable-write(w662, w661, w660) -> (w663:refnum<k21>, w664:errorcluster)  [unwired: 1 in, 1 out]
          }
          frame -2220 {
            n143 = Wait (ms)(milliseconds to wait=u32 10) -> ()  [unwired: 1 out]
          }
        }
        n144 = case shown="Error" w646 {
          selector: w646 -> [w654 w658]
          tunnel: [enum16{"Connect", "Send"}."Send" ("Message states") enum16{"Connect", "Send"}."Connect" ("Message states")] -> w645
          tunnel: [w654 errorcluster {"status"=FALSE, "code"=0, "source"=""} ("error IO")] -> w644
          tunnel: w643 -> [w652 w657]
          tunnel: [w652 w655] -> w642
          frame No Error {
          }
          frame Error {
            w655 = refnum<k21> refnum  # writer endpoint
            n145 = Destroy Stream Endpoint(8:w658, 11:w657) -> ()  [unwired: 1 out]
          }
        }
      }
    }
    n146 = shared-variable ".\\RT Variables.lvlib\\Stop RT Loops"() -> (w625:bool)  [unwired: 1 in, 1 out]
  }
  n147 = while {
    tunnel: [w670] -> w53
    shift-right: [w675] -> _
    shift-left: refnum<k21> refnum ("reader endpoint") -> [w673]
    shift-right: [w674] -> _
    shift-left: enum16{"Connect", "Receive"}."Connect" ("Message states") -> [w676]
    tunnel: w5 -> [w672]
    tunnel: w5 -> [w668]
    stop <- w669 stop-if-true
    # "Message loop"
    n148 = case shown="\"Receive\"" w676 {
      tunnel: [w683 w708] -> w671
      tunnel: [w681 w709] -> w675
      tunnel: [w690 w705] -> w674
      tunnel: w673 -> [_ w704]
      tunnel: w672 -> [_ w707]
      tunnel: [FALSE ("Stop RT Loops") w706] -> w669
      tunnel: w668 -> [_ w701]
      frame "Connect" {
        # "Attempts connection with the UI every 5 seconds, once successful, proceeds to Receive state."
        n149 = Bundle("", variant, variant) -> (w686:cluster{string, variant, variant})  [unwired: 1 in]
        n150 = Create Network Stream Reader Endpoint(5:5000 ("timeout in ms (-1)"), 7:4096 ("reader buffer size"), 9:w686, 11:"message reader" ("reader name")) -> (0:w685:errorcluster, 3:w680:refnum<k21>)  [unwired: 3 in]
        n151 = case shown="Error" w685 {
          selector: w685 -> [w695 _]
          tunnel: [enum16{"Connect", "Receive"}."Receive" ("Message states") enum16{"Connect", "Receive"}."Connect" ("Message states")] -> w690
          tunnel: [w694 errorcluster {"status"=FALSE, "code"=0, "source"=""} ("error IO")] -> w683
          tunnel: [w693 refnum<k21> refnum ("reader endpoint")] -> w681
          tunnel: w680 -> [w693 _]
          frame No Error {
            n152 = shared-variable ".\\RT Variables.lvlib\\2setpoint"(w693, error in=w695) -> (error out=w694:errorcluster)
          }
          frame Error {
          }
        }
      }
      frame "Receive" {
        # "Receives messages from the UI."
        n153 = shared-variable-read(w704, w707) -> (w703:refnum<k21>, w710:errorcluster, w700:cluster{string, variant, variant})  [unwired: 1 in, 1 out]
        n154 = Unbundle(w700) -> (w712:string, w711:variant, w702:variant)
        n155 = case shown="\"Vector Setpoints\"" w712 {
          tunnel: w711 -> [_ w733 w748 w754 w773]
          tunnel: w710 -> [w716 w735 w737 w753 w767]
          tunnel: [w715 w730 w744 w755 w763] -> w708
          tunnel: [refnum<k21> refnum ("reader endpoint") refnum<k21> refnum ("reader endpoint") w743 w761 w771] -> w709
          tunnel: w703 -> [w714 w729 w743 w761 w771]
          tunnel: [FALSE ("Stop RT Loops") w732 FALSE ("Stop RT Loops") FALSE ("Stop RT Loops") FALSE ("Stop RT Loops")] -> w706
          tunnel: [enum16{"Connect", "Receive"}."Connect" ("Message states") enum16{"Connect", "Receive"}."Receive" ("Message states") enum16{"Connect", "Receive"}."Receive" ("Message states") enum16{"Connect", "Receive"}."Receive" ("Message states") enum16{"Connect", "Receive"}."Receive" ("Message states")] -> w705
          tunnel: w702 -> [_ w725 w736 w757 w766]
          tunnel: w701 -> [_ w724 _ _ _]
          frame "Disconnect UI", Default {
            n156 = Destroy Stream Endpoint(8:w716, 11:w714) -> (0:w715:errorcluster)
          }
          frame "Stop" {
            n157 = Variant To Data(error in=w724, type=TRUE ("Stop RT Loops"), Variant=w725) -> (data=w722:bool, error out=w726:errorcluster)
            n158 = Variant To Data(error in=w735, type=TRUE ("Stop RT Loops"), Variant=w733) -> (data=w732:bool, error out=w734:errorcluster)
            n159 = shared-variable ".\\RT Variables.lvlib\\Stop RT Loops"(w732, error in=w734) -> (error out=w720:errorcluster)
            n160 = shared-variable ".\\RT Variables.lvlib\\Stop RT Loops"(w722, error in=w726) -> (error out=w721:errorcluster)
            n161 = Merge Errors(w720, w721) -> (w719:errorcluster)
            n162 = Destroy Stream Endpoint(8:w719, 11:w729) -> (0:w730:errorcluster)
          }
          frame "Update setpoint" {
            n163 = Variant To Data(error in=w737, type=0.0, Variant=w748) -> (data=w746:dbl, error out=w745:errorcluster)
            n164 = Variant To Data(error in=w737, type=0.0, Variant=w736) -> (data=w739:dbl, error out=w738:errorcluster)
            n165 = shared-variable ".\\RT Variables.lvlib\\Setpoint"(w746, error in=w745) -> (error out=w744:errorcluster)
            n166 = shared-variable ".\\RT Variables.lvlib\\Setpoint2"(w739, error in=w738) -> ()  [unwired: 1 out]
          }
          frame "Vector Setpoints" {
            n167 = Variant To Data(error in=w753, type=dbl[][][] [], Variant=w754) -> (data=w751:dbl[][][])  [unwired: 1 out]
            "vectores" <- w751
            n168 = Variant To Data(error in=w753, type=0.0, Variant=w757) -> (data=w756:dbl)  [unwired: 1 out]
            n169 = shared-variable ".\\RT Variables.lvlib\\Tiempo"(w756) -> (error out=w755:errorcluster)  [unwired: 1 in]
            n170 = Index Array(array=w751) -> (element #1=w750:dbl[][], element #2=w749:dbl[][])  [unwired: 6 in]
            "subarray" <- w750
            "subarray 2" <- w749
            n171 = shared-variable "myRIO-1900\\Untitled Library 7.lvlib\\subarray 2"(w749) -> ()  [unwired: 1 in, 1 out]
            n172 = shared-variable "myRIO-1900\\Untitled Library 6.lvlib\\subarray"(w750) -> ()  [unwired: 1 in, 1 out]
          }
          frame "Homing" {
            n173 = Variant To Data(error in=w767, type=TRUE, Variant=w773) -> (data=w765:bool, error out=w764:errorcluster)
            n174 = Variant To Data(error in=w767, type=0.0, Variant=w766) -> (data=→"data":dbl)  [unwired: 1 out]
            n175 = shared-variable ".\\RT Variables.lvlib\\Homing"(w765, error in=w764) -> (error out=w763:errorcluster)
          }
        }
      }
    }
    n176 = case shown="No Error" w671 {
      selector: w671 -> [w677 w678]
      tunnel: [w677 w678] -> w670
      frame No Error {
        # "No action required."
      }
      frame Error {
        # "Stops RT in case of error."
        n177 = shared-variable ".\\RT Variables.lvlib\\Stop RT Loops"(TRUE ("Stop RT Loops")) -> ()  [unwired: 1 in, 1 out]
      }
    }
  }
  n178 = Destroy Stream Endpoint(8:w57, 11:w56) -> (0:w54:errorcluster)
  n179 = node-c288(w60) -> ()  [unwired: 1 out]
  n180 = case shown="Error" w49 {
    selector: w49 -> [w774 w775]
    tunnel: [w774 w775] -> w11
    frame No Error {
      # "No action required."
    }
    frame Error {
      # "Destroys Message network stream to stop Message loop, in case of error."
      n181 = shared-variable ".\\RT Variables.lvlib\\2setpoint"() -> (w776:refnum<k21>)  [unwired: 1 in, 1 out]
      n182 = Destroy Stream Endpoint(11:w776) -> ()  [unwired: 1 in, 1 out]
    }
  }
  n183 = call <vilib>:"Stop.vi"("error in (no error)"=w11, "Encoder Ref In"=w41) -> ("error out"=w42:errorcluster, "Encoder Ref Out"=w43:T10)  [unwired: 8 in]
  n184 = call <vilib>:"Stop.vi"("error in (no error)"=w11, "Encoder Ref In"=w10) -> ("error out"=w13:errorcluster, "Encoder Ref Out"=w14:T10)  [unwired: 8 in]
  n185 = call <vilib>:"Close.vi"("error in (no error)"=w42, "Encoder Ref In"=w43) -> ("error out"=w36:errorcluster)  [unwired: 9 in]
  n186 = call <vilib>:"Close.vi"("error in (no error)"=w13, "Encoder Ref In"=w14) -> ("error out"=w12:errorcluster)  [unwired: 9 in]
  n187 = call <vilib>:"Close.vi"("error in (no error)"=w36, "PWM Ref In"=w33) -> ("error out"=w35:errorcluster)  [unwired: 9 in]
  n188 = call <vilib>:"Close.vi"("error in (no error)"=w12, "PWM Ref In"=w9) -> ("error out"=w8:errorcluster)  [unwired: 9 in]
  n189 = Merge Errors(w54, w53, w35, w8) -> (w52:errorcluster)
  n190 = shared-variable "myRIO-1900\\Network Shared Variables.lvlib\\error IO"(w52) -> ()  [unwired: 1 in, 1 out]
